vi "PH_O2_Watch.evt Set Limit.vi"(0 "i ref in":refnum<vi>, 2 "O2 Watch Instance":string="N/A", 3 "Limit [%]":dbl, 5 "error in (no error)":errorcluster) -> (14 "i ref out":refnum<vi>, 19 "error out":errorcluster)   [LabVIEW 2014, in "PH_O2_Watch.lvlib"]
doc: "This VI sends a \"SetLimit\" to the connected O2 Watch device."
uses:
  PH_O2_Watch.lvlib
  CSCore/CSSystem/CoreLib/CoreLib.double 2 byte array.vi
  CSCore/BaseProcess/BaseProcess.lvlib
  CSCore/CSSystem/CoreLib/CoreLib.lvlib
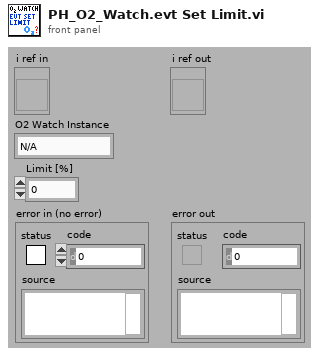
[diagram p1: front panel]
types:
  T1 = typedef "CoreDefs.rawDataType.ctl" = i8[]
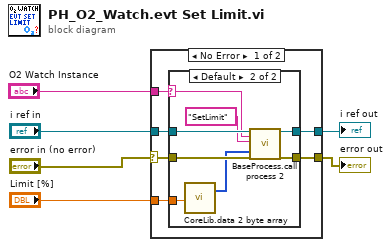
[diagram p0: block diagram]
diagram:
  n1 = case shown="No Error" "error in (no error)" {
    selector: "error in (no error)" -> [w8 w23]
    tunnel: [w12 w24] -> w6
    tunnel: [w11 w23] -> w5
    tunnel: "i ref in" -> [w10 w24]
    tunnel: "O2 Watch Instance" -> [w9 _]
    tunnel: "Limit [%]" -> [w7 _]
    frame No Error {
      n2 = case shown="Default" w9 {
        selector: w9 -> [_ w19]
        tunnel: [w14 w22] -> w12
        tunnel: [w13 w17] -> w11
        tunnel: w10 -> [w14 w21]
        tunnel: w8 -> [w13 w18]
        tunnel: w7 -> [_ w16]
        frame "N/A" {
        }
        frame Default {
          n3 = call-poly "CoreLib.data 2 byte array.vi"("f64"=w16) -> ("byteArray out"=w15:T1)  [unwired: 18 in]
          n4 = call "BaseProcess.call process 2.vi"("i ref in"=w21, "Object"=w19, "Selector"="SetLimit", "Data"=w15, "error in (no error)"=w18) -> ("i ref out"=w22:refnum<vi>, "error out"=w17:errorcluster)  [unwired: 13 in]
        }
      }
    }
    frame Error {
    }
  }
  "error out" <- w5
  "i ref out" <- w6
